vi "Echo QDFunction.vi"(0 "QDList":refnum<class "QDDialogList.lvclass">, 1 "Shift Pressed?":bool, 5 "QD Launch VI Ref":refnum<vi>, 7 "QD Combo Box Ref":refnum<vi>, 9 "QDFunction":string, 11 "error in (no error)":errorcluster, 12 "Variant in":variant) -> (4 "QDList":refnum<class "QDDialogList.lvclass">, 15 "error out":errorcluster)   [LabVIEW 2015, in "QDDialogList.lvclass"]
uses:
  QDDialogList.lvclass
  QDDialogList.lvclass/QDDialogList.ctl
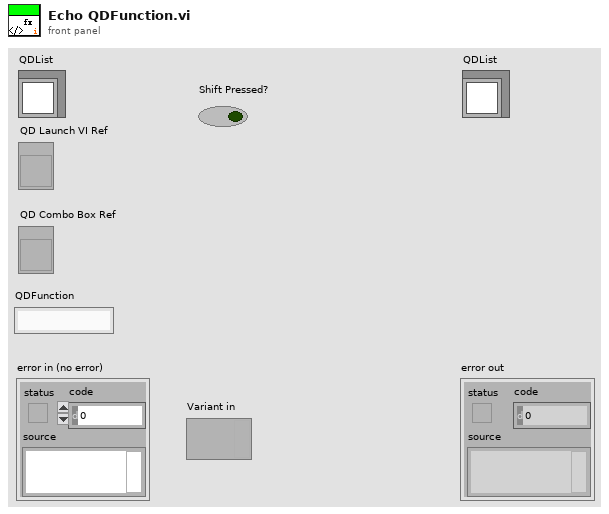
[diagram p1: front panel]
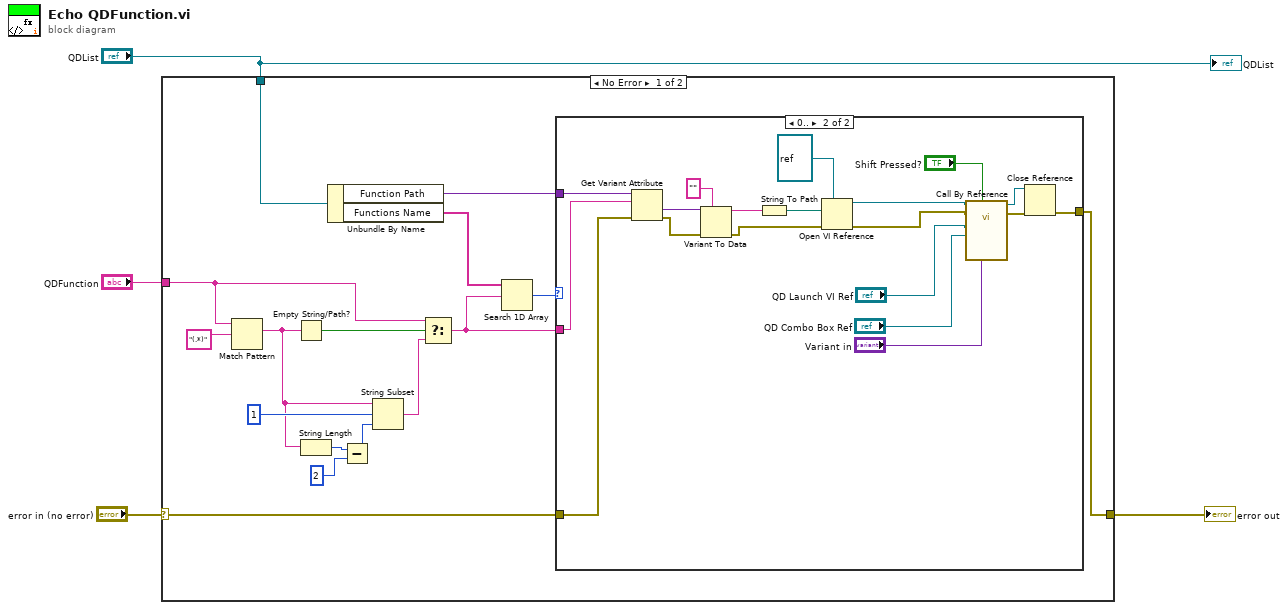
[diagram p0: block diagram]
diagram:
  n1 = case shown="No Error" "error in (no error)" {
    selector: "error in (no error)" -> [w7 w41]
    tunnel: "QDFunction" -> [w18 _]
    tunnel: [w6 w41] -> w2
    tunnel: "QDList" -> [w5 _]
    frame No Error {
      n2 = Match Pattern(string=w18, regular expression="(.*)") -> (match substring=w16:string)  [unwired: 1 in, 3 out]
      n3 = Empty String/Path?(string/path=w16) -> (empty?=w19:bool)
      n4 = String Length(string=w16) -> (length=w15:i32)
      n5 = Unbundle By Name(w5) -> ("Function Path"=w9:variant, "Functions Name"=w11:string[])
      n6 = Subtract(x=w15, y=2) -> (x-y=w13:i32)
      n7 = String Subset(string=w16, offset (0)=1, length (rest)=w13) -> (substring=w12:string)
      n8 = Select(t=w18, s=w19, f=w12) -> (s? t:f=w8:string)
      n9 = Search 1D Array(1D array=w11, element=w8) -> (index of element=w10:i32)  [unwired: 1 in]
      n10 = case shown="0.." w10 {
        tunnel: w9 -> [_ w38]
        tunnel: w8 -> [_ w37]
        tunnel: w7 -> [w21 w33]
        tunnel: [w21 w23] -> w6
        frame Default {
        }
        frame 0.. {
          n11 = Get Variant Attribute(Variant=w38, name=w37, error in=w33) -> (value=w36:variant, error out=w34:errorcluster)  [unwired: 1 in, 2 out]
          n12 = Variant To Data(error in=w34, type="", Variant=w36) -> (data=w32:string, error out=w31:errorcluster)
          n13 = String To Path(string=w32) -> (path=w40:path)
          n14 = Open VI Reference(type specifier VI Refnum (for type only)=refnum<vi> refnum, vi path=w40, error in (no error)=w31) -> (vi reference=w30:refnum<vi>, error out=w29:errorcluster)  [unwired: 3 in]
          n15 = call-by-ref "?"(reference=w30, error in=w29, "Variant in"="Variant in", "Shift Pressed?"="Shift Pressed?", "QD Combo Box Ref"="QD Combo Box Ref", "QD Launch VI Ref"="QD Launch VI Ref") -> (reference out=w22:refnum<vi>, error out=w24:errorcluster)  [unwired: 6 in, 2 out]
          n16 = Close Reference(reference=w22, error in (no error)=w24) -> (error out=w23:errorcluster)
        }
      }
    }
    frame Error {
    }
  }
  "error out" <- w2
  "QDList" <- "QDList"
